vi "write_elements_rates.vi"(0 "Elements + Rates":cluster{"Elements":u16[], "Rates":sgl[]} {"Rates" format="%_4f"; "Elements" items=["None", "Ag", "AgBr", "AgCl", "Al", "Al2O3", "Al4C3", "AlF3", "AlN", "AlSb", "As", "As2Se3", "Au", "B", "B2O3", "B4C", "BN", "Ba", "BaF2", "BaN2O6", "BaO", "BaTiO3", "BaTiO3", "Be", "BeF2", "BeO", "Bi", "Bi2O3", "Bi2S3", "Bi2Se3", "Bi2Te3", "BiF3", "C", "C", "C8H8", "Ca", "CaF2", "CaO", "CaO-SiO2", "CaSO4", "CaTiO3", "CaWO4", "Cd", "CdF2", "CdO", "CdS", "CdSe", "CdTe", "Ce", "CeF3", "CeO2", "Co", "CoO", "Cr", "Cr2O3", "Cr3C2", "CrB", "Cs", "Cs2SO4", "CsBr", "CsCI", "CsI", "Cu", "Cu2O", "Cu2S", "Cu2S", "CuS", "Dy", "DY2O3", "Er", "Er2O3", "Eu", "EuF2", "Fe", "Fe2O3", "FeO", "FeS", "Ga", "Ga2O3", "GaAs", "GaN", "GaP", "GaSb", "Gd", "Gd2O3", "Ge", "Ge3N2", "GeO2", "GeTe", "Hf", "HfB2", "HfC", "HfN", "HfO2", "HfSi2", "Hg", "Ho", "Ho2O3", "In", "In2O3", "In2Se3", "In2Te3", "InAs", "InP", "InSb", "Ir", "K", "KBr", "KCI", "KF", "KI", "La", "La2O3", "LaB6", "LaF3", "Li", "LiBr", "LiF", "LiNbO3", "Lu", "Mg", "MgAl2O4", "MgAl2O6", "MgF2", "MgO", "Mn", "MnO", "MnS", "Mo", "Mo2C", "MoB2", "MoO3", "MoS2", "Na", "Na3AIF6", "Na5Al3F14", "NaBr", "NaCl", "NaCIO3", "NaF", "NaNO3", "Nb", "Nb2O3", "Nb2O5", "NbB2", "NbC", "NbN", "Nd", "Nd2O3", "NdF3", "Ni", "NiCr", "NiCrFe", "NiFe", "NiFeMo", "NiO", "P3N5", "Pb", "PbCl2", "PbF2", "PbO", "PbS", "PbSe", "PbSnO3", "PbTe", "Pd", "PdO", "Po", "Pr", "Pr2O3", "Pt", "PtO2", "Ra", "Rb", "RbI", "Re", "Rh", "Ru", "S8", "Sb", "Sb2O3", "Sb2S3", "Sc", "Sc2O3", "Se", "Si", "Si3N4", "SiC", "SiO", "SiO2", "Sm", "Sm2O3", "Sn", "SnO2", "SnS", "SnSe", "SnTe", "Sr", "SrF2", "SrO", "Ta", "Ta2O5", "TaB2", "TaC", "TaN", "Tb", "Tc", "Te", "TeO2", "Th", "ThF4", "ThO2", "ThOF2", "Ti", "Ti2O3", "TiB2", "TiC", "TiN", "TiO", "TiO2", "TI", "TIBr", "TICI", "TII", "U", "U3O8", "U4O9", "UO2", "V", "V2O5", "VB2", "VC", "VN", "VO2", "W", "WB2", "WC", "WO3", "WS2", "WSi2", "Y", "Y2O3", "Yb", "Yb2O3", "Zn", "Zn3Sb2", "ZnF2", "ZnO", "ZnS", "ZnSe", "ZnTe", "Zr", "ZrB2", "ZrC", "ZrN", "ZrO2"]}) -> ()   [LabVIEW 2012]
panel:
  out "Response":string
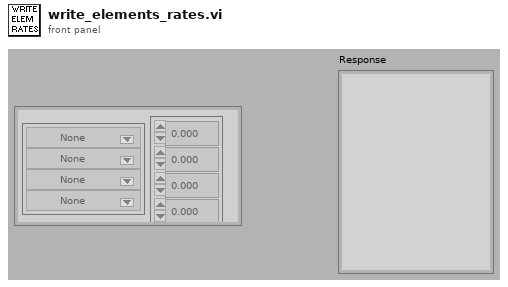
[diagram p1: front panel]
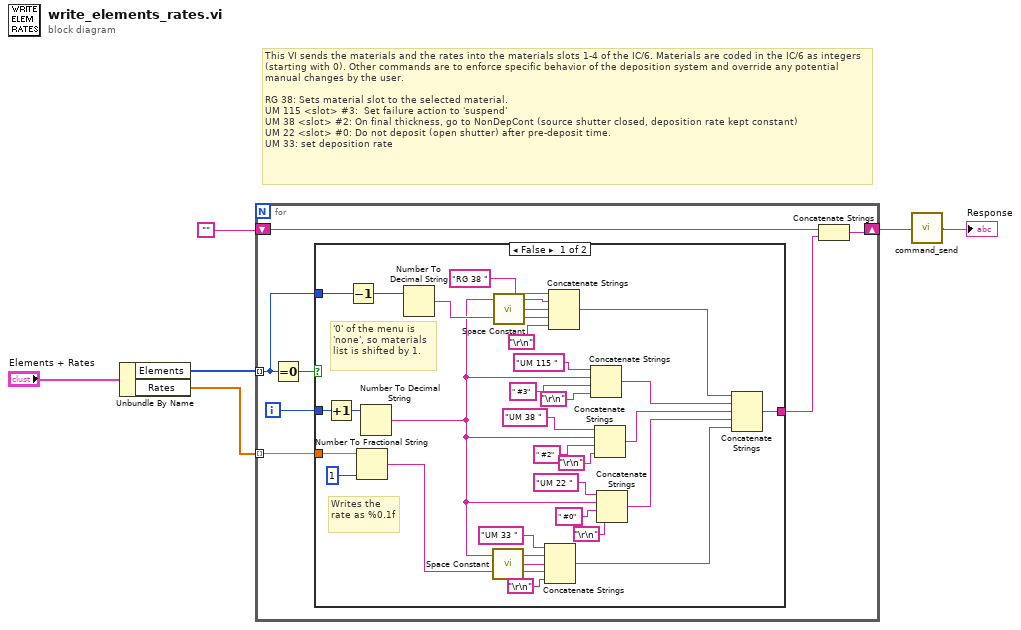
[diagram p0: block diagram]
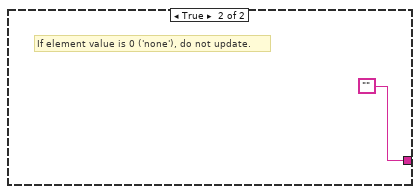
[diagram p2: hidden frame]
diagram:
  # "This VI sends the materials and the rates into the materials slots 1-4 of the IC/6. Materials are coded in the IC/6 as integers (starting with 0). Other commands are to enforce specific behavior of the deposition system and override any potential manual changes by the user.\n\nRG 38: Sets material slot to the selected material.\nUM 115 <slot> #3:  Set failure action to 'suspend'\nUM 38 <slot> #2: On final thickness, go to NonDepCont (source shutter closed, deposition rate kept constant)\nUM 22 <slot> #0: Do not deposit (open shutter) after pre-deposit time.\nUM 33: set deposition rate"
  n1 = Unbundle By Name("Elements + Rates") -> ("Elements"=w6:u16[], "Rates"=w5:sgl[])
  n2 = for {
    tunnel: w6 -> [w12] mode=indexing
    tunnel: w5 -> [w11] mode=indexing
    shift-right: [w8] -> w1
    shift-left: "" -> [w9]
    i -> [w10]
    n3 = Equal To 0?(x=w12) -> (x = 0?=w13:bool)
    n4 = case shown="False" w13 {
      tunnel: w12 -> [w43 _]
      tunnel: w11 -> [w42 _]
      tunnel: w10 -> [w36 _]
      tunnel: [w35 ""] -> w7
      frame False {
        # "'0' of the menu is 'none', so materials list is shifted by 1."
        # "Writes the rate as %0.1f"
        n5 = Increment(x=w36) -> (x+1=w37:i32)
        n6 = Decrement(x=w43) -> (x-1=w41:u16)
        n7 = Number To Fractional String(number=w42, precision (6)=1) -> (F-format string=w32:string)  [unwired: 2 in]
        n8 = Number To Decimal String(number=w37) -> (decimal integer string=w20:string)  [unwired: 1 in]
        n9 = Number To Decimal String(number=w41) -> (decimal integer string=w33:string)  [unwired: 1 in]
        n10 = call <vilib>:"Space Constant.vi"() -> ("String"=w31:string)
        n11 = call <vilib>:"Space Constant.vi"() -> ("String"=w38:string)
        n12 = Concatenate Strings("UM 33 ", w20, w31, w32, "\r\n") -> (w28:string)
        n13 = Concatenate Strings("RG 38 ", w20, w38, w33, "\r\n") -> (w17:string)
        n14 = Concatenate Strings("UM 115 ", w20, " #3", "\r\n") -> (w16:string)
        n15 = Concatenate Strings("UM 38 ", w20, " #2", "\r\n") -> (w14:string)
        n16 = Concatenate Strings("UM 22 ", w20, " #0", "\r\n") -> (w15:string)
        n17 = Concatenate Strings(w17, w16, w14, w15, w28) -> (w35:string)
      }
      frame True {
        # "If element value is 0 ('none'), do not update."
      }
    }
    n18 = Concatenate Strings(w9, w7) -> (w8:string)
  }
  n19 = call "command_send.vi"("Commands"=w1) -> ("Response"=→"Response":string)
